vi "Periodic Tasks.vi"(8 "Error In":errorcluster) -> ()   [LabVIEW 2012]
doc: "This VI runs in parallel to other tasks. It can contain as many user-defined periodic loops as you need. These can carry out PID or other sorts of timed response."
uses:
  Globals/Potentiometers.vi
  Globals/Robot Jaguars.vi
  Globals/DriveSystemMode.vi
  <vilib>/Rock Robotics/WPI/Joystick/WPI_JoystickGetSetRefNum.vi
  Globals/Calculated Shooter Speed.vi
  Globals/Image Height.vi
  Globals/Alignment Error.vi
  Globals/Drive Commands.vi
  Globals/Load Cell Multiplier.vi
panel:
  out "Peak for Shooter":dbl
  in  "Peak End (Commit)":dbl
  in  "Peak Start":dbl
  out "IR":bool
  in  "Reset Max Value":bool
  in  "Ball Offset":dbl
  out "Driver Multiplier":dbl=0.9944881889763779
  out "Load Cell Multiplier":dbl=1.0
  out "Load Cell":dbl=0.5385810950000001
  out "Sensor Plot":dbl(graph)=0.5385810950000001
  out "Load Cell Max Value":dbl=0.554001806
  in  "Throttle Raw":dbl=0.11023622047244094
  out "axis 3 (throttle)":dbl=0.11023622047244094
  in  "Post speed gain":dbl=0.23
  out "Center of Mass X 2":dbl(graph)=298.96
  in  "reinitialize? (F)":bool=TRUE
  out "Raw String from UDP":string="!195,298.96,173.18,132.00,92.00,461.31,366.92,129.00,105.00,143.32,371.39,129.00,97.00,#END"
  out "Aiming Error":dbl=-21.04000000000002
  in  "Center of Mass X":dbl=298.96
  in  "Invert":bool=TRUE
  in  "PID gains":T1={"proportional gain (Kc)"=0.0076, "integral time (Ti, min)"=0.0, "derivative time (Td, min)"=0.0031} {"derivative time (Td, min)" format="%.6f"; "integral time (Ti, min)" format="%.9f"; "proportional gain (Kc)" format="%.6f"}
  in  "PID gains (actuator)":T1={"proportional gain (Kc)"=1.95, "integral time (Ti, min)"=0.0, "derivative time (Td, min)"=0.0} {"derivative time (Td, min)" format="%.6f"; "integral time (Ti, min)" format="%.3f"; "proportional gain (Kc)" format="%.3f"}
  in  "PID gains (weak motor)":T1={"proportional gain (Kc)"=8.0, "integral time (Ti, min)"=0.0, "derivative time (Td, min)"=0.0} {"derivative time (Td, min)" format="%.6f"; "integral time (Ti, min)" format="%.3f"; "proportional gain (Kc)" format="%.3f"}
  in  "PID gains (strong motor)":T1={"proportional gain (Kc)"=4.0, "integral time (Ti, min)"=0.0, "derivative time (Td, min)"=0.0} {"derivative time (Td, min)" format="%.6f"; "integral time (Ti, min)" format="%.3f"; "proportional gain (Kc)" format="%.3f"}
  # "Steers"
  # "Steering"
  # "Actuator"
  # "Shooter"
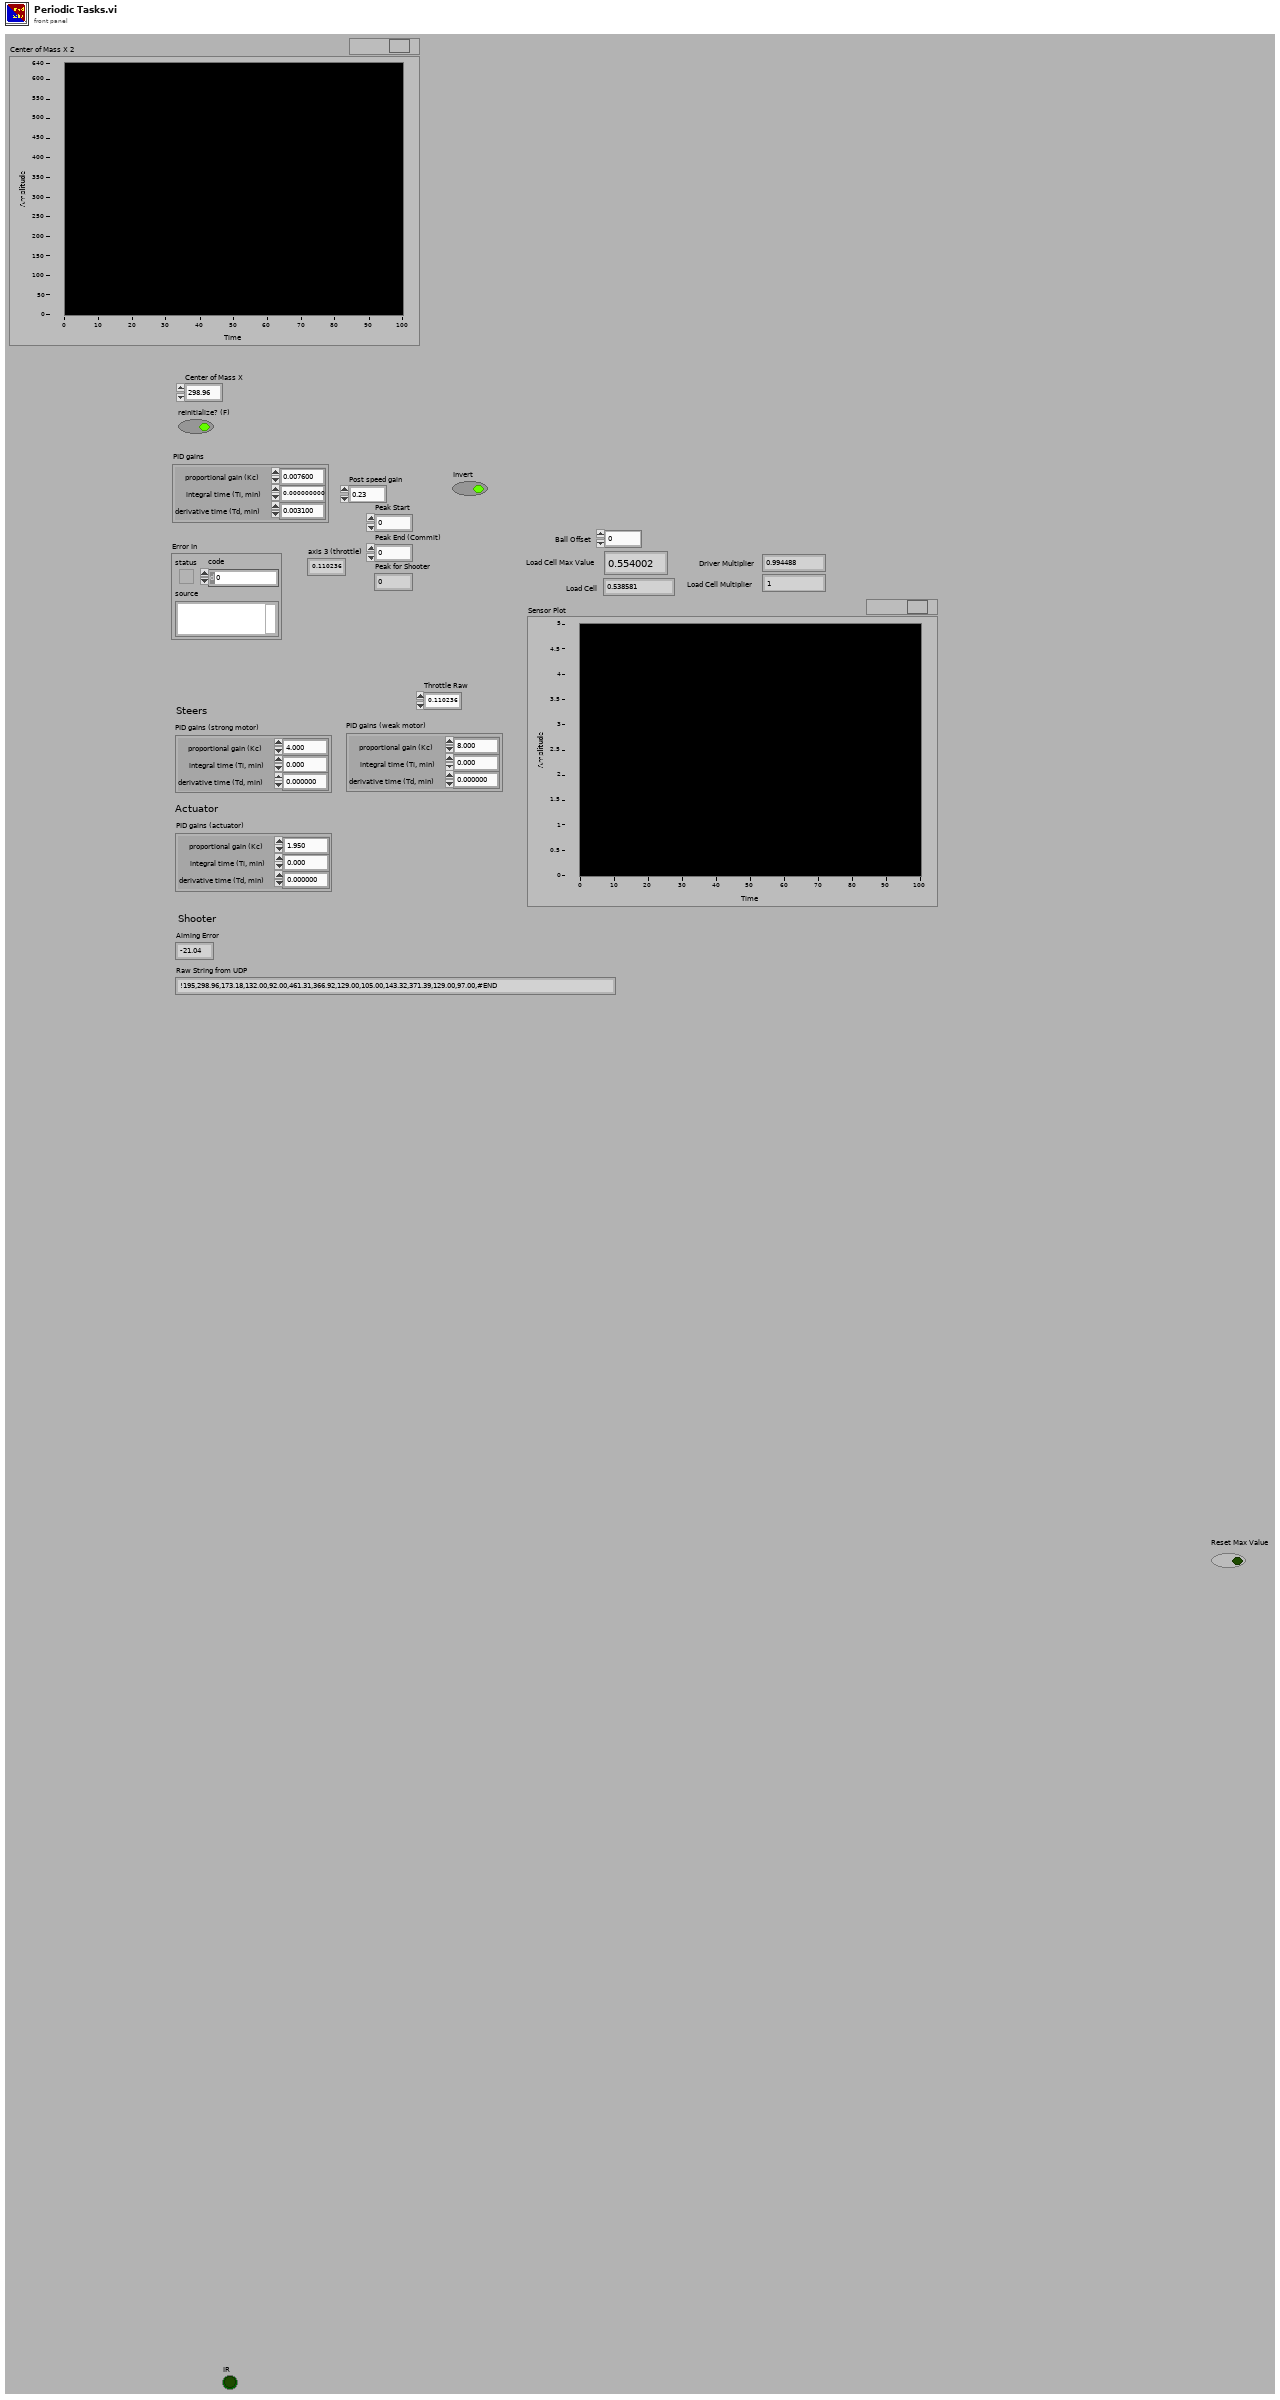
[diagram p1: front panel]
types:
  T1 = cluster{"proportional gain (Kc)":dbl, "integral time (Ti, min)":dbl, "derivative time (Td, min)":dbl}
  T2 = cluster{"Front Left Drive":dbl, "Front Right Drive":dbl, "Rear Left Drive":dbl, "Rear Right Drive":dbl, "Front Left Steer":dbl, "Front Right Steer":dbl, "Rear Left Steer":dbl, "Rear Right Steer":dbl}
  T3 = typedef "WPI_AnalogChannelDevRef.ctl" = cluster{"DevStatus":errorcluster, "Analog Module":T4, "Analog Channel":T5}
  T4 = typedef "FPGA_TypedefAnalogModule.ctl" = enum16{"Analog Module 1", "Analog Module 2"}
  T5 = typedef "FPGA_AIChannel.ctl" = enum8{"AI 1", "AI 2", "AI 3", "AI 4", "AI 5", "AI 6", "AI 7", "AI 8", "Invalid"}
  T6 = typedef "WPI_DigitalInputDevRef.ctl" = cluster{"DevStatus":errorcluster, "DIO Channel":T7, "Digital Module":T8}
  T7 = typedef "FPGA_DIOChannel.ctl" = enum8{"DIO 1", "DIO 2", "DIO 3", "DIO 4", "DIO 5", "DIO 6", "DIO 7", "DIO 8", "DIO 9", "DIO 10", "DIO 11", "DIO 12", "DIO 13", "DIO 14", "Invalid"}
  T8 = typedef "FPGA_TypedefDigitalModule.ctl" = enum16{"Digital Module 1", "Digital Module 2"}
  T9 = typedef "WPI_JoystickDevRef.ctl" = cluster{"Device":T10}
  T10 = typedef "WPI_JoystickDeviceEnum.ctl" = enum16{"USB 1", "USB 2", "USB 3", "USB 4", "Kinect 1", "Kinect 2"}
  T11 = typedef "WPI_JoystickButtonState.ctl" = cluster{"Button 1":bool, "Button 2":bool, "Button 3":bool, "Button 4":bool, "Button 5":bool, "Button 6":bool, "Button 7":bool, "Button 8":bool, "Button 9":bool, "Button 10":bool, "Button 11":bool, "Button 12":bool}
  T12 = typedef "Drive System Mode.ctl" = enum16{"Normal", "Crab", "Shoot"}
  T13 = cluster{"Front Left":T3, "Front Right":T3, "Rear Left":T3, "Rear Right":T3, "Actuator":T3}
  T14 = typedef "WPI_MotorControlDeviceRef.ctl" = cluster{"DeviceStatus":errorcluster, "Type":enum16{"PWM", "CAN"}, "PWM":cluster{"Digital Module":T8, "PWM Channel":T15, "DeadBand":T16}, "CAN":cluster{"Device Number":u8, "Control Mode":T17, "Semaphore":T18, "Max Vout":dbl}, "Invert":bool, "TransformRef":T19, "InvTransformRef":T19}
  T15 = typedef "FPGA_DIOPWMChannel.ctl" = enum8{"PWM 1", "PWM 2", "PWM 3", "PWM 4", "PWM 5", "PWM 6", "PWM 7", "PWM 8", "PWM 9", "PWM 10", "Invalid"}
  T16 = typedef "WPI_PWMDeadband.ctl" = cluster{"Name":string, "maxPositivePwm":i32, "minPositivePwm":i32, "centerPwm":i32, "maxNegativePwm":i32, "minNegativePwm":i32, "angularRange":u16}
  T17 = typedef "WPI_CANJaguar_ControlMode.ctl" = enum8{"Percent VBus", "Current", "Speed", "Position", "Voltage"}
  T18 = typedef "Semaphore RefNum" = refnum<k1>
  T19 = typedef "WPI_PWMTransform_ConPane.ctl" = refnum<vi>
  T20 = cluster{"Front Left Drive":T14, "Front Right Drive":T14, "Rear Left Drive":T14, "Rear Right Drive":T14, "Front Left Steer":T14, "Front Right Steer":T14, "Rear Left Steer":T14, "Rear Right Steer":T14}
  T21 = typedef "WPI_GyroDevRef.ctl" = cluster{"DevStatus":errorcluster, "Analog Module":T4, "Analog Channel":T5, "Offset":dbl, "Gain (VoltsPerDegree/Second)":dbl}
  T22 = cluster{"axis 1 (x)":dbl, "axis 2 (y)":dbl, "axis 3 (throttle)":dbl, "axis 4":dbl, "axis 5":dbl, "axis 6":dbl}
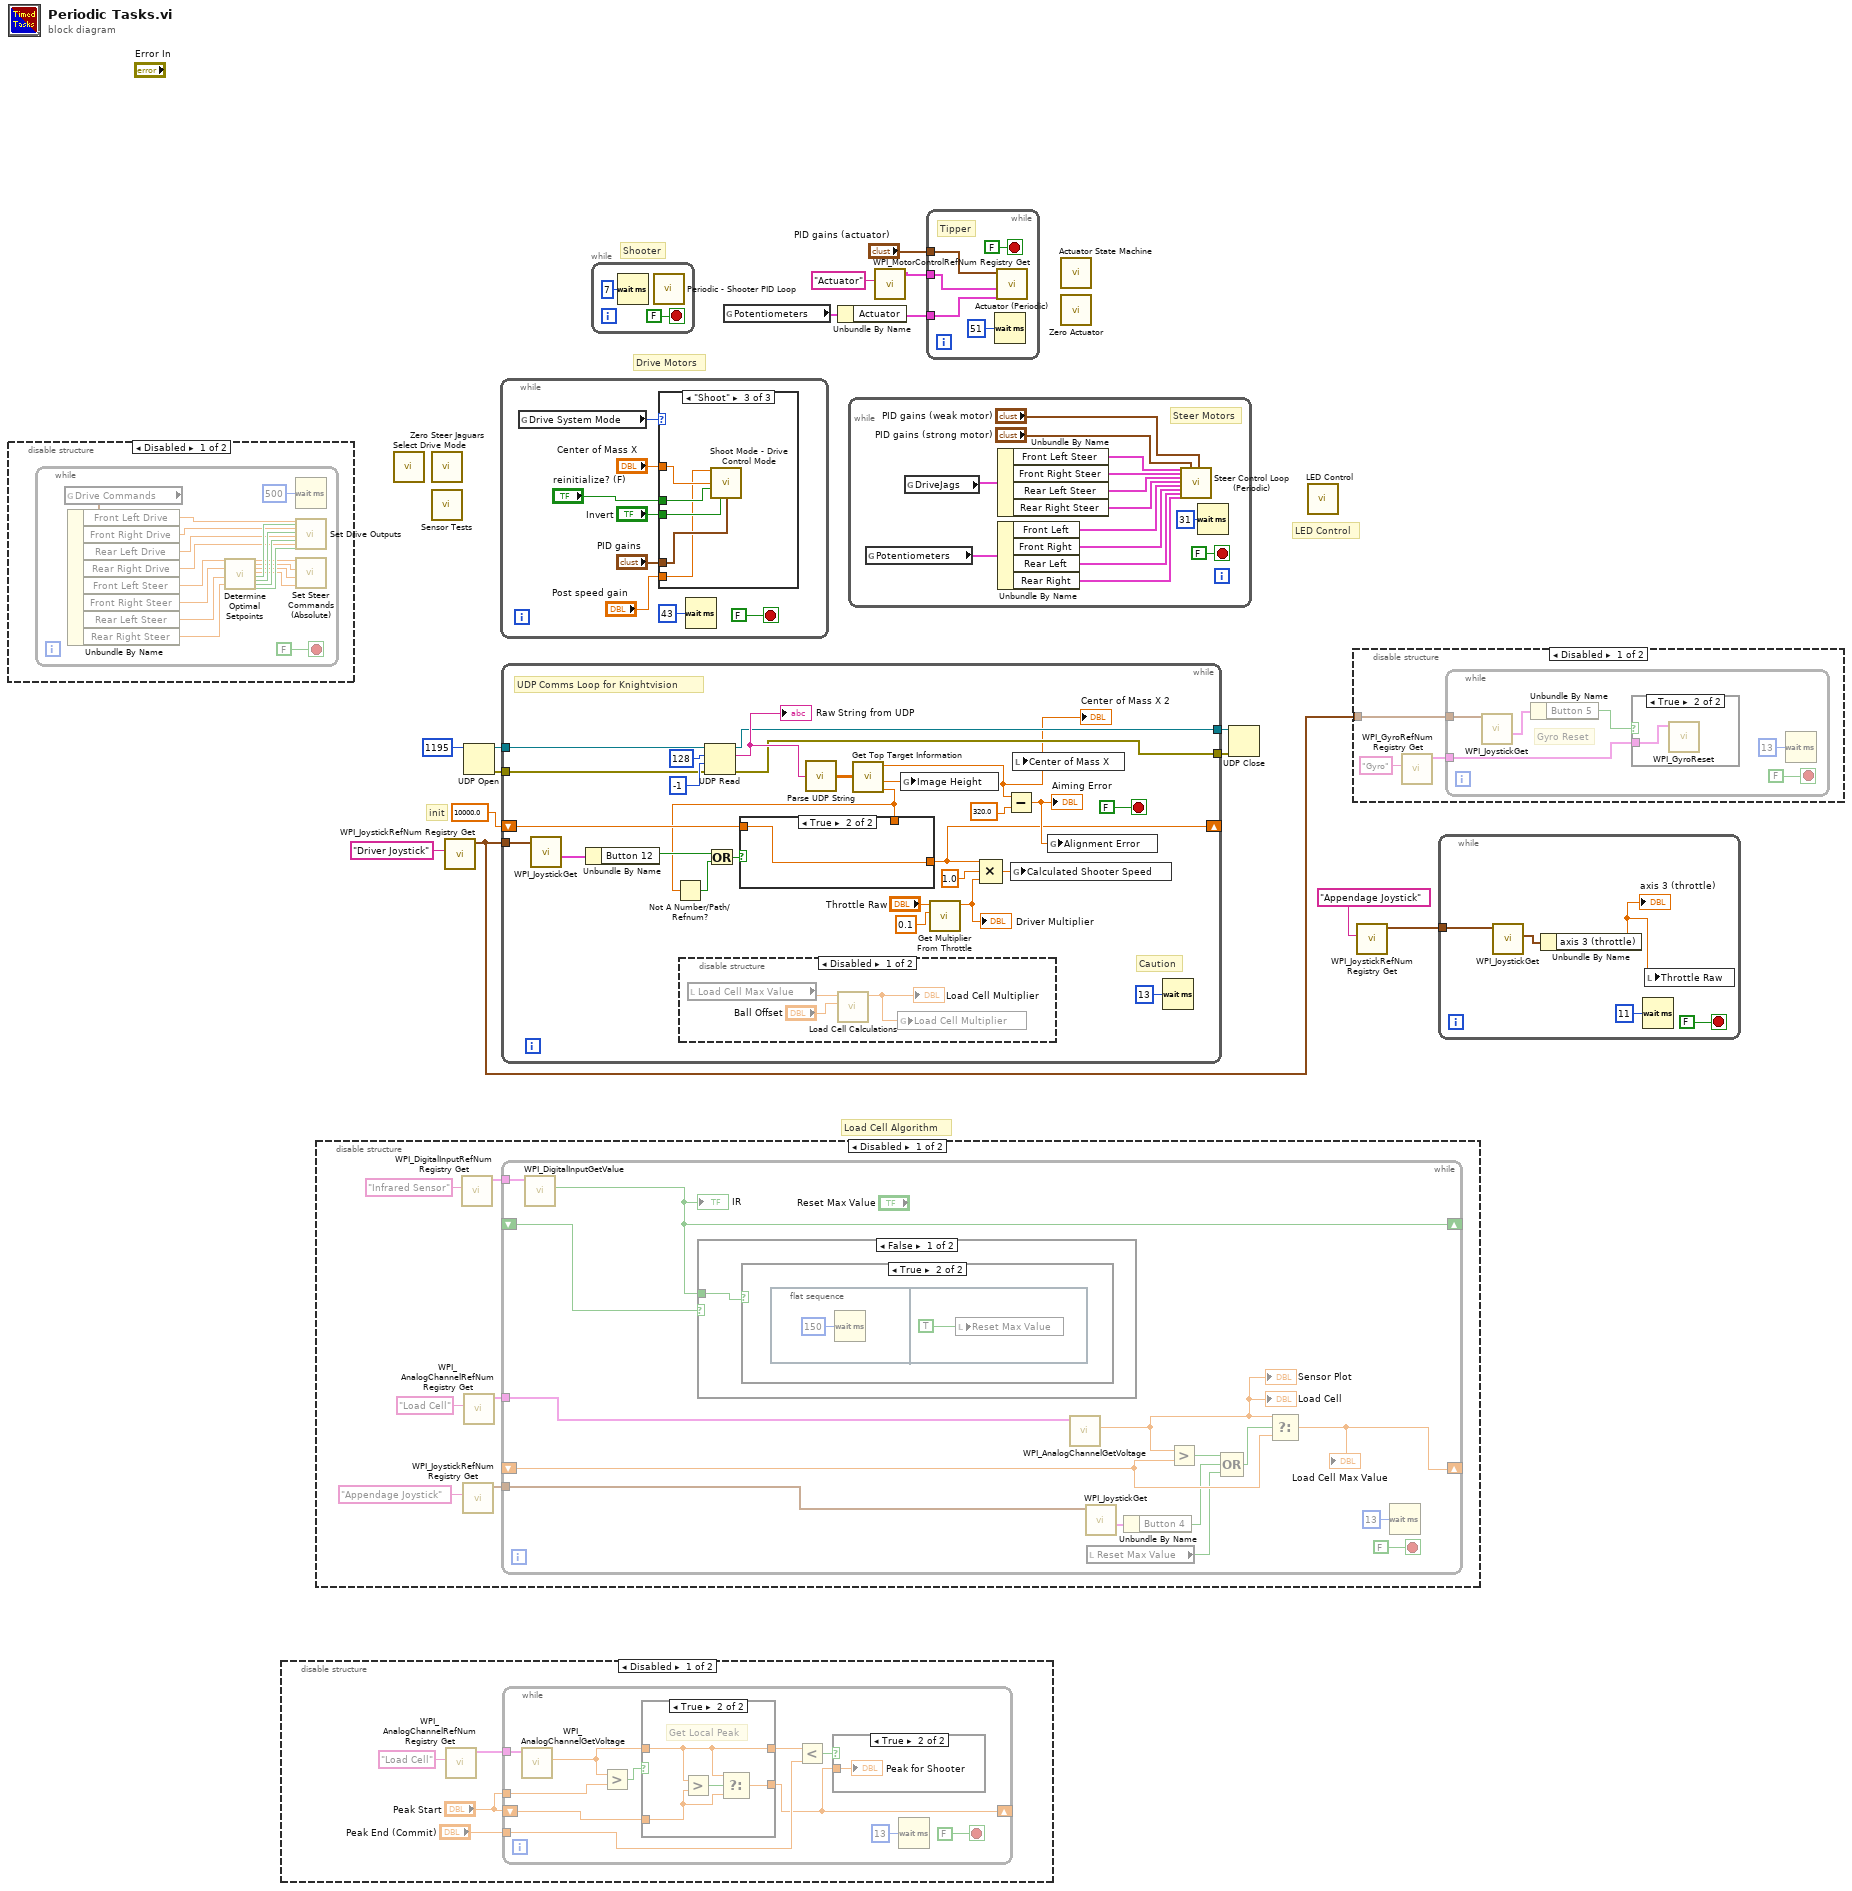
[diagram p0: block diagram]
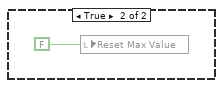
[diagram p6: hidden frame]
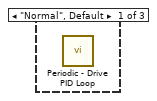
[diagram p8: hidden frame]
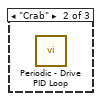
[diagram p9: hidden frame]
diagram:
  # "LED Control"
  # "Drive Motors"
  # "Shooter"
  # "Load Cell Algorithm"
  # "init"
  n1 = disable-structure shown="Disabled" {
    frame Disabled {
      n2 = while {
        stop <- FALSE stop-if-true
        n3 = global read "Drive Commands.vi" "Drive Commands"() -> (w26:T2)
        n4 = Unbundle By Name(w26) -> ("Front Left Drive"=w25:dbl, "Front Right Drive"=w24:dbl, "Rear Left Drive"=w23:dbl, "Rear Right Drive"=w22:dbl, "Front Left Steer"=w21:dbl, "Front Right Steer"=w20:dbl, "Rear Left Steer"=w19:dbl, "Rear Right Steer"=w18:dbl)
        n5 = call "Determine Optimal Setpoints.vi"("Front Left"=w21, "Front Right"=w20, "Rear Left"=w19, "Rear Right"=w18) -> ("Front Left Out"=w30:dbl, "Front Right Out"=w29:dbl, "Rear Left Out"=w28:dbl, "Rear Right Out"=w27:dbl, "Inv. Front Left Drive?"=w31:bool, "Inv. Front Right Drive?"=w32:bool, "Inv. Rear Left Drive?"=w33:bool, "Inv. Rear Right Drive?"=w34:bool)  [unwired: 16 in]
        n6 = Wait (ms)(milliseconds to wait=u32 500) -> ()  [unwired: 1 out]
        n7 = call "Set Drive Outputs.vi"("Front Left"=w25, "Inv Front Left"=w31, "Front Right"=w24, "Inv Front Right"=w32, "Rear Left"=w23, "Inv Rear Left"=w33, "Rear Right"=w22, "Inv Rear Right"=w34) -> ()  [unwired: 20 in]
        n8 = call "Set Steer Commands (Absolute).vi"("Rear Right"=w27, "Rear Left"=w28, "Front Right"=w29, "Front Left"=w30) -> ()  [unwired: 8 in]
      }
    }
    frame Enabled {
    }
  }
  n9 = disable-structure shown="Disabled" {
    frame Disabled {
      n10 = call <vilib>:"WPI_AnalogChannelRefNum Registry Get.vi"("refnum name"="Load Cell") -> ("AIDeviceRef"=w37:T3)  [unwired: 9 in, 1 out]
      n11 = while {
        tunnel: w37 -> [w49]
        tunnel: "Peak Start" -> [w48]
        shift-right: [w39] -> _
        shift-left: "Peak Start" -> [w44]
        tunnel: "Peak End (Commit)" -> [w43]
        stop <- FALSE stop-if-true
        n12 = call <vilib>:"WPI_AnalogChannelGetVoltage.vi"("AIDeviceRef"=w49) -> ("Voltage"=w42:dbl)  [unwired: 8 in, 2 out]
        n13 = Greater?(x=w42, y=w48) -> (0:w47:bool)
        n14 = case shown="True" w47 {
          tunnel: w42 -> [w51 w53]
          tunnel: [w52 w55] -> w39
          tunnel: w44 -> [w52 w54]
          tunnel: [w51 w53] -> w41
          frame False {
          }
          frame True {
            # "Get Local Peak"
            n15 = Greater?(x=w53, y=w54) -> (0:w56:bool)
            n16 = Select(t=w53, s=w56, f=w54) -> (s? t:f=w55:dbl)
          }
        }
        n17 = Less?(x=w41, y=w43) -> (x < y?=w40:bool)
        n18 = case shown="True" w40 {
          tunnel: w39 -> [_ w50]
          frame False {
            # "Keep current peak \nfor shooter"
          }
          frame True {
            "Peak for Shooter" <- w50
          }
        }
        n19 = Wait (ms)(milliseconds to wait=u32 13) -> ()  [unwired: 1 out]
      }
    }
    frame Enabled {
    }
  }
  n20 = disable-structure shown="Disabled" {
    frame Disabled {
      n21 = call <vilib>:"WPI_DigitalInputRefNum Registry Get.vi"("refnum name"="Infrared Sensor") -> ("DigitalInputDevRef"=w57:T6)  [unwired: 9 in, 1 out]
      n22 = call <vilib>:"WPI_JoystickRefNum Registry Get.vi"("refnum name"="Appendage Joystick") -> ("JoystickDevRef"=w59:T9)  [unwired: 9 in, 1 out]
      n23 = call <vilib>:"WPI_AnalogChannelRefNum Registry Get.vi"("refnum name"="Load Cell") -> ("AIDeviceRef"=w61:T3)  [unwired: 9 in, 1 out]
      n24 = while {
        tunnel: w61 -> [w77]
        shift-right: [w69] -> _
        shift-left: _ -> [w74]
        tunnel: w59 -> [w72]
        tunnel: w57 -> [w67]
        shift-right: [w65] -> _
        shift-left: _ -> [w66]
        stop <- FALSE stop-if-true
        n25 = call <vilib>:"WPI_DigitalInputGetValue.vi"("DigitalInputDevRef"=w67) -> ("Value"=w65:bool)  [unwired: 8 in, 2 out]
        "IR" <- w65
        n26 = case shown="False" w66 {
          tunnel: w65 -> [w78 _]
          frame False {
            n27 = case shown="True" w78 {
              frame False {
              }
              frame True {
                n28 = flat-sequence {
                  frame #0 {
                    n29 = Wait (ms)(milliseconds to wait=u32 150) -> ()  [unwired: 1 out]
                  }
                  frame #1 {
                    n30 = local write "Reset Max Value"(TRUE ("Reset Load Cell Value")) -> ()
                  }
                }
              }
            }
          }
          frame True {
            n31 = local write "Reset Max Value"(FALSE ("Reset Load Cell Value")) -> ()
          }
        }
        n32 = call <vilib>:"WPI_AnalogChannelGetVoltage.vi"("AIDeviceRef"=w77) -> ("Voltage"=w68:dbl)  [unwired: 8 in, 2 out]
        "Sensor Plot" <- w68
        "Load Cell" <- w68
        n33 = call <vilib>:"WPI_JoystickGet.vi"("JoystickDevRef"=w72) -> ("Buttons"=w71:T11)  [unwired: 4 in, 2 out]
        n34 = local read "Reset Max Value"() -> (w64:bool)
        n35 = Unbundle By Name(w71) -> ("Button 4"=w63:bool)
        n36 = Greater?(x=w68, y=w74) -> (0:w73:bool)
        n37 = Compound Arithmetic op=OR(w73, w63, w64) -> (w70:bool)
        n38 = Select(t=w68, s=w70, f=w74) -> (s? t:f=w69:dbl)
        "Load Cell Max Value" <- w69
        n39 = Wait (ms)(milliseconds to wait=u32 13) -> ()  [unwired: 1 out]
      }
    }
    frame Enabled {
    }
  }
  n40 = call "Select Drive Mode.vi"() -> ()  [unwired: 12 in]
  n41 = call "Zero Steer Jaguars.vi"() -> ()  [unwired: 12 in]
  n42 = call "Sensor Tests.vi"() -> ()  [unwired: 12 in]
  n43 = call <vilib>:"WPI_JoystickRefNum Registry Get.vi"("refnum name"="Driver Joystick") -> ("JoystickDevRef"=w6:T9)  [unwired: 9 in, 1 out]
  n44 = UDP Open(11:u16 1195 ("port")) -> (port=w14:refnum<k16>, 0:w13:errorcluster)  [unwired: 4 in, 1 out]
  n45 = while {
    stop <- FALSE stop-if-true
    n46 = global read "DriveSystemMode.vi" "Drive System Mode"() -> (w87:T12)
    n47 = case shown="\"Shoot\"" w87 {
      tunnel: "PID gains" -> [_ _ w94]
      tunnel: "Invert" -> [_ _ w93]
      tunnel: "Center of Mass X" -> [_ _ w92]
      tunnel: "reinitialize? (F)" -> [_ _ w91]
      tunnel: "Post speed gain" -> [_ _ w90]
      frame "Normal", Default {
        n48 = call "Periodic - Drive PID Loop.vi"() -> ()  [unwired: 12 in]
      }
      frame "Crab" {
        n49 = call "Periodic - Drive PID Loop.vi"() -> ()  [unwired: 12 in]
      }
      frame "Shoot" {
        n50 = call "Shoot Mode - Drive Control Mode.vi"("Post Speed Limit"=w90, "Center of Mass X"=w92, "reinitialize? (F)"=w91, "Invert"=w93, "PID gains"=w94) -> ()  [unwired: 11 in]
      }
    }
    n51 = Wait (ms)(milliseconds to wait=u32 43) -> ()  [unwired: 1 out]
  }
  n52 = while {
    tunnel: w14 -> [w115]
    tunnel: w13 -> [w114]
    tunnel: [w113] -> w12
    tunnel: [w112] -> w11
    shift-right: [w100] -> _
    shift-left: 10000.0 ("Calculated Shooter Speed") -> [w110]
    tunnel: w6 -> [w108]
    stop <- FALSE stop-if-true
    # "Caution"
    # "UDP Comms Loop for Knightvision"
    n53 = call <vilib>:"WPI_JoystickGet.vi"("JoystickDevRef"=w108) -> ("Buttons"=w109:T11)  [unwired: 4 in, 2 out]
    n54 = Unbundle By Name(w109) -> ("Button 12"=w105:bool)
    n55 = disable-structure shown="Disabled" {
      frame Disabled {
        n56 = local read "Load Cell Max Value"() -> (w124:dbl)
        n57 = call "Load Cell Calculations.vi"("Ball Offset"="Ball Offset", "Load Cell Value"=w124) -> ("Multiplier"=w122:dbl)  [unwired: 9 in]
        "Load Cell Multiplier" <- w122
        n58 = global write "Load Cell Multiplier.vi" "Load Cell Multiplier"(w122) -> ()
      }
      frame Enabled {
      }
    }
    n59 = UDP Read(connection ID=w115, max size (548)=128, timeout ms (25000)=-1, 8:w114) -> (data out=w120:string, error out=w112:errorcluster, 3:w113:refnum<k16>)  [unwired: 2 out]
    "Raw String from UDP" <- w120
    n60 = call "Parse UDP String.vi"("UDP Packet In"=w120) -> ("Array"=w117:dbl[][])
    n61 = call "Get Top Target Information.vi"("Vision Info Array"=w117) -> ("Center of Mass X"=w111:dbl, "Bounding Box Height"=w106:dbl, "Calculated Shooter Speed"=w103:dbl)  [unwired: 1 out]
    "Center of Mass X 2" <- w111
    n62 = Not A Number/Path/Refnum?(number/path/refnum=w103) -> (NaN/Path/Refnum?=w102:bool)
    n63 = Or(x=w105, y=w102) -> (x .or. y?=w104:bool)
    n64 = case shown="True" w104 {
      tunnel: w103 -> [w125 _]
      tunnel: [w125 w126] -> w100
      tunnel: w110 -> [_ w126]
      frame False {
      }
      frame True {
      }
    }
    n65 = global write "Image Height.vi" "Image Height"(w106) -> ()
    n66 = call "Get Multiplier From Throttle.vi"("Value from 1"=0.1 ("y"), "Axis 3"="Throttle Raw") -> ("Numeric"=w95:dbl)  [unwired: 9 in]
    "Driver Multiplier" <- w95
    n67 = Compound Arithmetic op=MULTIPLY(w100, 1.0 ("value"), w95) -> (w101:dbl)
    n68 = Subtract(x=w111, y=320.0) -> (x-y=w107:dbl)
    "Aiming Error" <- w107
    n69 = global write "Calculated Shooter Speed.vi" "Calculated Shooter Speed"(w101) -> ()
    n70 = local write "Center of Mass X"(w111) -> ()
    n71 = global write "Alignment Error.vi" "Alignment Error"(w107) -> ()
    n72 = Wait (ms)(milliseconds to wait=u32 13) -> ()  [unwired: 1 out]
  }
  n73 = while {
    stop <- FALSE stop-if-true
    n74 = Wait (ms)(milliseconds to wait=u32 7) -> ()  [unwired: 1 out]
    n75 = call "Periodic - Shooter PID Loop.vi"() -> ()  [unwired: 1 in]
  }
  n76 = global read "Potentiometers.vi" "Potentiometers"() -> (w5:T13)
  n77 = Unbundle By Name(w5) -> ("Actuator"=w2:T3)
  n78 = while {
    stop <- FALSE stop-if-true
    # "Steer Motors"
    n79 = global read "Potentiometers.vi" "Potentiometers"() -> (w139:T13)
    n80 = global read "Robot Jaguars.vi" "DriveJags"() -> (w140:T20)
    n81 = Unbundle By Name(w140) -> ("Front Left Steer"=w138:T14, "Front Right Steer"=w137:T14, "Rear Left Steer"=w136:T14, "Rear Right Steer"=w135:T14)
    n82 = Unbundle By Name(w139) -> ("Front Left"=w134:T3, "Front Right"=w133:T3, "Rear Left"=w132:T3, "Rear Right"=w131:T3)
    n83 = call "Steer Control Loop (Periodic).vi"("Front Left Steer"=w138, "Front Right Steer"=w137, "Rear Left Steer"=w136, "Rear Right Steer"=w135, "Front Left Pot"=w134, "Front Right Pot"=w133, "Rear Left Pot"=w132, "Rear Right Pot"=w131, "PID gains (strong motor)"="PID gains (strong motor)", "PID gains (weak motor)"="PID gains (weak motor)") -> ()  [unwired: 18 in]
    n84 = Wait (ms)(milliseconds to wait=u32 31) -> ()  [unwired: 1 out]
  }
  n85 = call <vilib>:"WPI_MotorControlRefNum Registry Get.vi"("refnum name"="Actuator") -> ("MotorControlDevRef"=w3:T14)  [unwired: 9 in, 1 out]
  n86 = while {
    tunnel: w3 -> [w145]
    tunnel: w2 -> [w144]
    tunnel: "PID gains (actuator)" -> [w143]
    stop <- FALSE stop-if-true
    # "Tipper"
    n87 = Wait (ms)(milliseconds to wait=u32 51) -> ()  [unwired: 1 out]
    n88 = call "Actuator (Periodic).vi"("Pot"=w144, "Motor"=w145, "PID gains (actuator)"=w143) -> ()  [unwired: 8 in, 1 out]
  }
  n89 = call "Actuator State Machine.vi"() -> ()  [unwired: 1 in]
  n90 = call "Zero Actuator.vi"() -> ()  [unwired: 12 in]
  n91 = UDP Close(connection ID=w12, 8:w11) -> ()  [unwired: 2 out]
  n92 = call "LED Control.vi"() -> ()  [unwired: 12 in]
  n93 = disable-structure shown="Disabled" {
    disable-tunnel: w6 -> [w148 _]
    frame Disabled {
      n94 = call <vilib>:"WPI_GyroRefNum Registry Get.vi"("refnum name"="Gyro") -> ("GyroDevRef"=w149:T21)  [unwired: 9 in, 1 out]
      n95 = while {
        tunnel: w148 -> [w153]
        tunnel: w149 -> [w151]
        stop <- FALSE stop-if-true
        # "Gyro Reset"
        n96 = call <vilib>:"WPI_JoystickGet.vi"("JoystickDevRef"=w153) -> ("Buttons"=w154:T11)  [unwired: 4 in, 2 out]
        n97 = Unbundle By Name(w154) -> ("Button 5"=w152:bool)
        n98 = case shown="True" w152 {
          tunnel: w151 -> [_ w157]
          frame False {
          }
          frame True {
            n99 = call <vilib>:"WPI_GyroReset.vi"("GyroDevRef"=w157) -> ()  [unwired: 9 in, 2 out]
          }
        }
        n100 = Wait (ms)(milliseconds to wait=u32 13) -> ()  [unwired: 1 out]
      }
    }
    frame Enabled {
    }
  }
  n101 = call <vilib>:"WPI_JoystickRefNum Registry Get.vi"("refnum name"="Appendage Joystick") -> ("JoystickDevRef"=w8:T9)  [unwired: 9 in, 1 out]
  n102 = while {
    tunnel: w8 -> [w161]
    stop <- FALSE stop-if-true
    n103 = call <vilib>:"WPI_JoystickGet.vi"("JoystickDevRef"=w161) -> ("Axes"=w162:T22)  [unwired: 4 in, 2 out]
    n104 = Unbundle By Name(w162) -> ("axis 3 (throttle)"=w158:dbl)
    "axis 3 (throttle)" <- w158
    n105 = Wait (ms)(milliseconds to wait=u32 11) -> ()  [unwired: 1 out]
    n106 = local write "Throttle Raw"(w158) -> ()
  }
